vi "OutputControl.vi"(8 "error in (no error)":errorcluster, 10 "On":bool, 11 "RMX4120 in":refnum<class "RMX4120.lvclass">) -> (0 "error out":errorcluster, 3 "RMX4120 out":refnum<class "RMX4120.lvclass">)   [LabVIEW 2023, in "RMX4120.lvclass"]
uses:
  RMX4120.lvclass
  RMXPowerSupply.lvclass
panel:
  # "True:On\nFalse:Off"
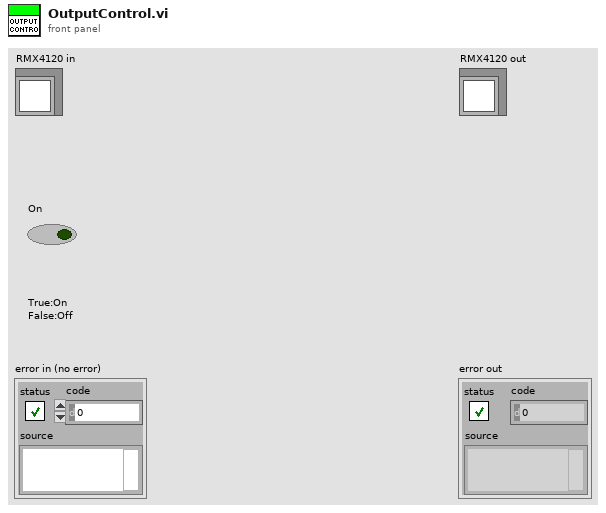
[diagram p1: front panel]
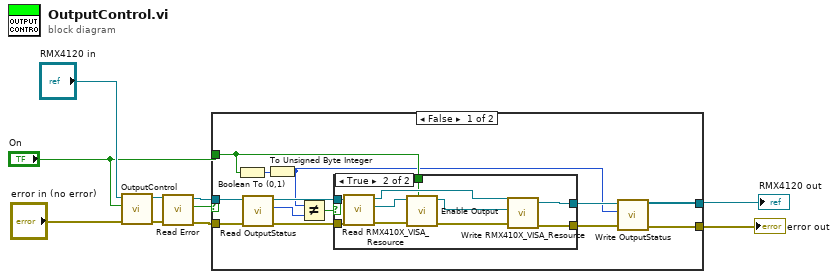
[diagram p0: block diagram]
diagram:
  n1 = call-parent "OutputControl.vi"("error in (no error)"="error in (no error)", "On"="On", "RMXPowerSupply in"="RMX4120 in") -> ("error out"=w4:errorcluster, "RMXPowerSupply out"=w5:refnum<class "RMX4120.lvclass">)  [unwired: 7 in]
  n2 = call-dynamic "Read Error.vi"("error in (no error)"=w4, "RMXPowerSupply in"=w5) -> ("error out"=w3:errorcluster, "Error"=w1:bool, "RMXPowerSupply out"=w2:refnum<class "RMX4120.lvclass">)  [unwired: 7 in]
  n3 = case shown="False" w1 {
    tunnel: "On" -> [w14 _]
    tunnel: [w21 w36] -> w7
    tunnel: [w20 w37] -> w6
    tunnel: w3 -> [w18 w36]
    tunnel: w2 -> [w19 w37]
    frame False {
      n4 = Boolean To (0,1)(Boolean=w14) -> (0, 1=w15:i16)
      n5 = call-dynamic "Read OutputStatus.vi"("error in (no error)"=w18, "RMXPowerSupply in"=w19) -> ("error out"=w17:errorcluster, "OutputStatus"=w12:u8, "RMXPowerSupply out"=w16:refnum<class "RMX4120.lvclass">)  [unwired: 7 in]
      n6 = To Unsigned Byte Integer(number=w15) -> (unsigned 8bit integer=w13:u8)
      n7 = Not Equal?(x=w13, y=w12) -> (x != y?=w11:bool)
      n8 = case shown="True" w11 {
        tunnel: [w25 w30] -> w23
        tunnel: [w24 w29] -> w22
        tunnel: w17 -> [w24 w28]
        tunnel: w16 -> [w25 w27]
        tunnel: w14 -> [_ w26]
        frame False {
        }
        frame True {
          n9 = call-dynamic "Read RMX410X_VISA_Resource.vi"("error in (no error)"=w28, "RMXPowerSupply in"=w27) -> ("error out"=w34:errorcluster, "RMX410X_VISA_Resource"=w35:refnum<visa-resource-name>, "RMXPowerSupply out"=w32:refnum<class "RMX4120.lvclass">)  [unwired: 7 in]
          n10 = call "Enable Output.vi"("Enable Output (F: Disable)"=w26, "error in (no error)"=w34, "VISA resource name"=w35) -> ("error out"=w33:errorcluster, "VISA resource name out"=w31:refnum<visa-resource-name>)  [unwired: 7 in]
          n11 = call-dynamic "Write RMX410X_VISA_Resource.vi"("error in (no error)"=w33, "RMX410X_VISA_Resource"=w31, "RMXPowerSupply in"=w32) -> ("error out"=w29:errorcluster, "RMXPowerSupply out"=w30:refnum<class "RMX4120.lvclass">)  [unwired: 7 in]
        }
      }
      n12 = call-dynamic "Write OutputStatus.vi"("error in (no error)"=w22, "OutputStatus"=w13, "RMXPowerSupply in"=w23) -> ("error out"=w21:errorcluster, "RMXPowerSupply out"=w20:refnum<class "RMX4120.lvclass">)  [unwired: 7 in]
    }
    frame True {
    }
  }
  "error out" <- w7
  "RMX4120 out" <- w6
